vi "TEMPERATURE_TRANSMITTER.vi"(2 "Lower setpoint":dbl, 3 "Input":dbl, 4 "Higher setpoint":dbl) -> (0 "LOW":bool, 1 "HIGH":bool)   [LabVIEW 2014]
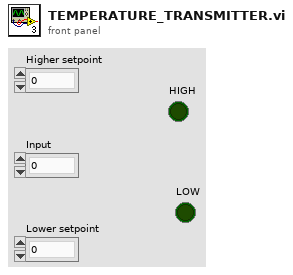
[diagram p1: front panel]
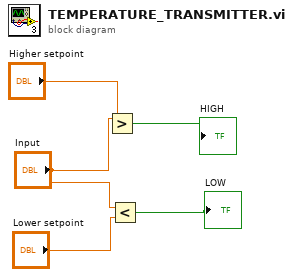
[diagram p0: block diagram]
diagram:
  n1 = Greater?(x="Input", y="Higher setpoint") -> (0:→"HIGH":bool)
  n2 = Less?(x="Input", y="Lower setpoint") -> (x < y?=→"LOW":bool)
